vi "LVPortPumpMessages.vi"(8 "error in":errorcluster, 11 "pID":string) -> (0 "error out":errorcluster, 3 "Created Event Count":i32)   [LabVIEW 2017]
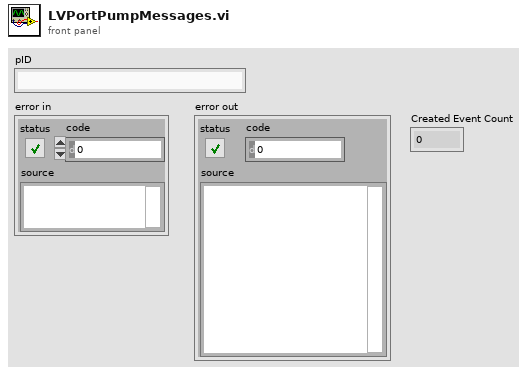
[diagram p1: front panel]
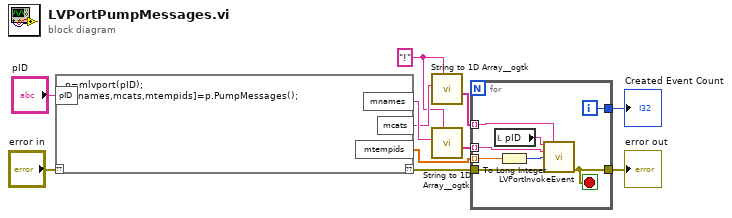
[diagram p0: block diagram]
diagram:
  w8 = "!" ("delimiter (Tab)")
  n1 = script code="p=mlvport(pID);\n[mnames,mcats,mtempids]=p.PumpMessages();"("??"="error in", "pID"="pID") -> ("??"=w3:errorcluster, "mnames"=w10:string, "mcats"=w9:string, "mtempids"=w5:dbl[])
  n2 = call <userlib>:"String to 1D Array__ogtk.vi"("delimiter (Tab)"=w8, "string"=w9) -> ("Array of Strings"=w6:string[])  [unwired: 9 in]
  n3 = call <userlib>:"String to 1D Array__ogtk.vi"("delimiter (Tab)"=w8, "string"=w10) -> ("Array of Strings"=w7:string[])  [unwired: 9 in]
  n4 = for {
    tunnel: w7 -> [w17] mode=indexing
    tunnel: w6 -> [w18] mode=indexing
    tunnel: w5 -> [w19] mode=indexing
    tunnel: w3 -> [w14]
    tunnel: [w13] -> w2
    tunnel: [w12] -> w1
    i -> [w12]
    stop <- w13 stop-if-true
    n5 = local read "pID"() -> (w16:string)
    n6 = To Long Integer(number=w19) -> (32bit integer=w15:i32)
    n7 = call "LVPortInvokeEvent.vi"("ID"=w16, "Category"=w18, "name"=w17, "Data"=w15, "error in (no error)"=w14) -> ("error out"=w13:errorcluster)  [unwired: 10 in]
  }
  "error out" <- w2
  "Created Event Count" <- w1
